vi "KLEUREN.vi"() -> ()   [LabVIEW 2018]
panel:
  in  "stop":bool
  in  "digital out":bool[](array[boolean])
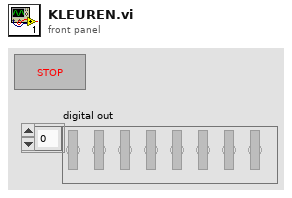
[diagram p1: front panel]
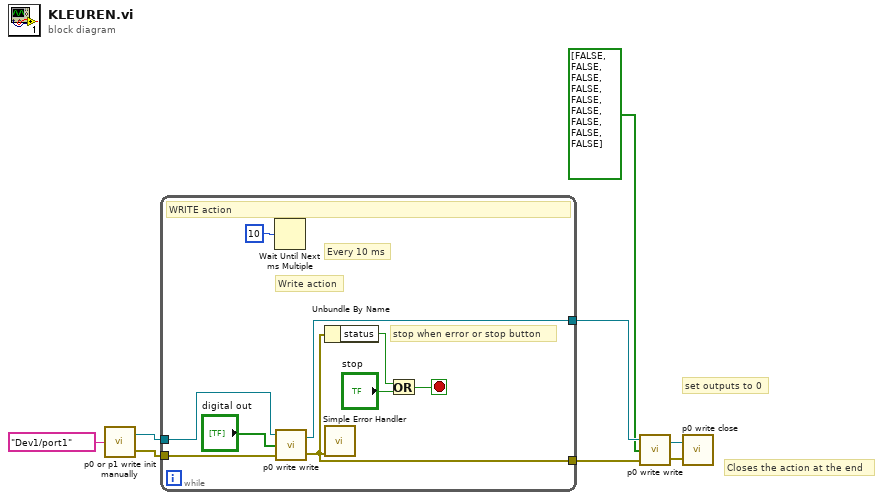
[diagram p0: block diagram]
diagram:
  # "set outputs to 0"
  # "Closes the action at the end"
  n1 = call "p0 or p1 write init manually.vi"("Port"=tag "Dev1/port1") -> ("task out"=w3:refnum<k21>, "error out"=w2:errorcluster)
  n2 = while {
    tunnel: w3 -> [w17]
    tunnel: [w16] -> w8
    tunnel: w2 -> [w15]
    tunnel: [w10] -> w7
    stop <- w11 stop-if-true
    # "stop when error or stop button"
    # "Every 10 ms"
    # "Write action"
    # "WRITE action"
    n3 = Wait Until Next ms Multiple(millisecond multiple=u32 10) -> ()  [unwired: 1 out]
    n4 = call "p0 write write.vi"("error in"=w15, "digital out"="digital out", "task/channels in"=w17) -> ("error out"=w10:errorcluster, "task out"=w16:refnum<k21>)
    n5 = Unbundle By Name(w10) -> ("status"=w9:bool)
    n6 = call <vilib>:"Simple Error Handler.vi"("error in (no error)"=w10) -> ()  [unwired: 4 in, 5 out]
    n7 = Or(x=w9, y="stop") -> (x .or. y?=w11:bool)
  }
  n8 = call "p0 write write.vi"("error in"=w7, "digital out"=bool[] [FALSE, FALSE, FALSE, FALSE, FALSE, FALSE, FALSE, FALSE, FALSE], "task/channels in"=w8) -> ("error out"=w5:errorcluster, "task out"=w6:refnum<k21>)
  n9 = call "p0 write close.vi"("error in"=w5, "task/channels in"=w6) -> ()
